vi "Update LS.vi"(8 "error in":errorcluster, 11 "PIOD in":refnum<class "PIOD.lvclass">) -> (0 "error out":errorcluster, 3 "PIOD out":refnum<class "PIOD.lvclass">)   [LabVIEW 2018, in "PIOD.lvlib" / "PIOD.lvclass"]
uses:
  PIOD.lvclass
  PPLs/PLC/Parent/PLC.lvlibp/PLC.lvclass
  C:/AME Test Engineering/LabVIEW/PPLs/PLC/Parent/PLC.lvlibp/PLC.lvclass
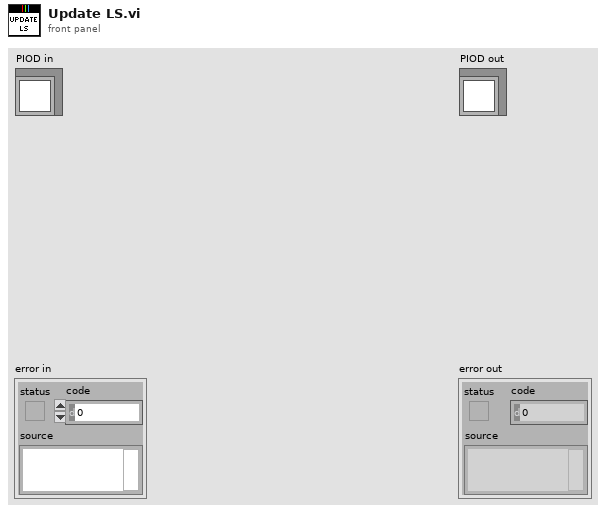
[diagram p1: front panel]
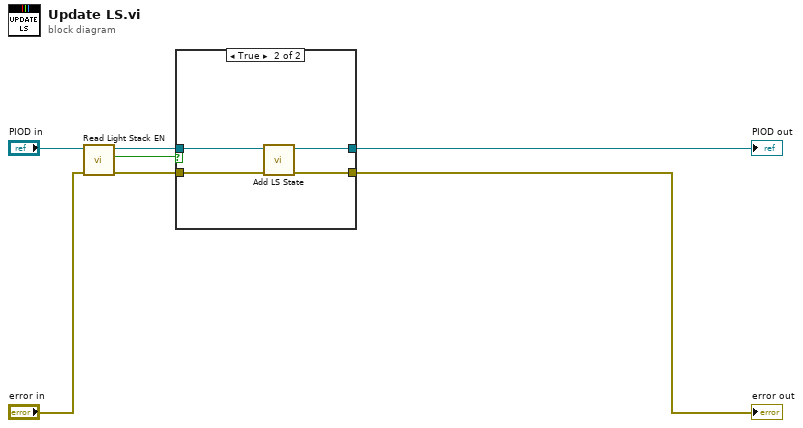
[diagram p0: block diagram]
diagram:
  n1 = call "Read Light Stack EN.vi"("error in (no error)"="error in", "PLC in"="PIOD in") -> ("error out"=w3:errorcluster, "Light Stack?"=w5:bool, "PLC out"=w4:refnum<class "PIOD.lvclass">)  [unwired: 7 in]
  n2 = case shown="True" w5 {
    tunnel: w4 -> [w9 w12]
    tunnel: w3 -> [w8 w13]
    tunnel: [w9 w11] -> w2
    tunnel: [w8 w10] -> w1
    frame False {
    }
    frame True {
      n3 = call "Add LS State.vi"("error in"=w13, "PIOD in"=w12) -> ("error out"=w10:errorcluster, "PIOD out"=w11:refnum<class "PIOD.lvclass">)  [unwired: 8 in]
    }
  }
  "error out" <- w1
  "PIOD out" <- w2
